vi "Plotter_Competition_Main_backup.vi"() -> ()   [LabVIEW 2014]
doc: "Buggy_Competition Main.vi\nv4.0\nCode fior Jan 2012\n\nModified by D.Readman 1/12/2011 to 5/1/2012 \n- Replaced shift registers with FGV's.\n- Latched Switch function added.\n- Digital filtering on encoder inputs added."
uses:
  Controls/Plotter States.ctl
  <vilib>/Platform/TimedLoop/XDataNode/timing_clust.ctl
  <vilib>/Platform/TimedLoop/XDataNode/nitl_modes.ctl
  <vilib>/Platform/TimedLoop/XDataNode/wakeup.ctl
  <vilib>/FPGAPlugInAG/myRIO-1900/niLvFpga_Open_myRIO-1900.vi
  <vilib>/rvi/interface/nirviOpenFPGA/nirviOpenFPGA.xnode
  FPGA Bitfiles/Buggycompetition_FPGATarget2_AeroBuggyFPGA_9DbUQD1BP7s.lvbitx
  FPGA/FPGA.vi
  <vilib>/Platform/TimedLoop/XDataNode/XDataNode.xnode
  <vilib>/Platform/TimedLoop/XDataNode/XDNodeRunTimeDep.lvlib
panel:
  out "Finished Late? [i-1]":bool
  in  "Sample interval":u32=100000
  in  "MWidth":i64=4
  out "Current State":T1
  out "Switch B":bool
  out "Switch A":bool
  in  "Enc. Filter":i16=2 min=0 step=1
  out "Switches Latched":cluster{"Switch A GN":bool, "Switch B BL":bool}
  in  "Terminate":bool
  out "Error Display":errorcluster
  in  "Reset Button":bool
  # "Impeccable Plotter Controller"
  # "Switches"
  # "Admin controls - Do not alter"
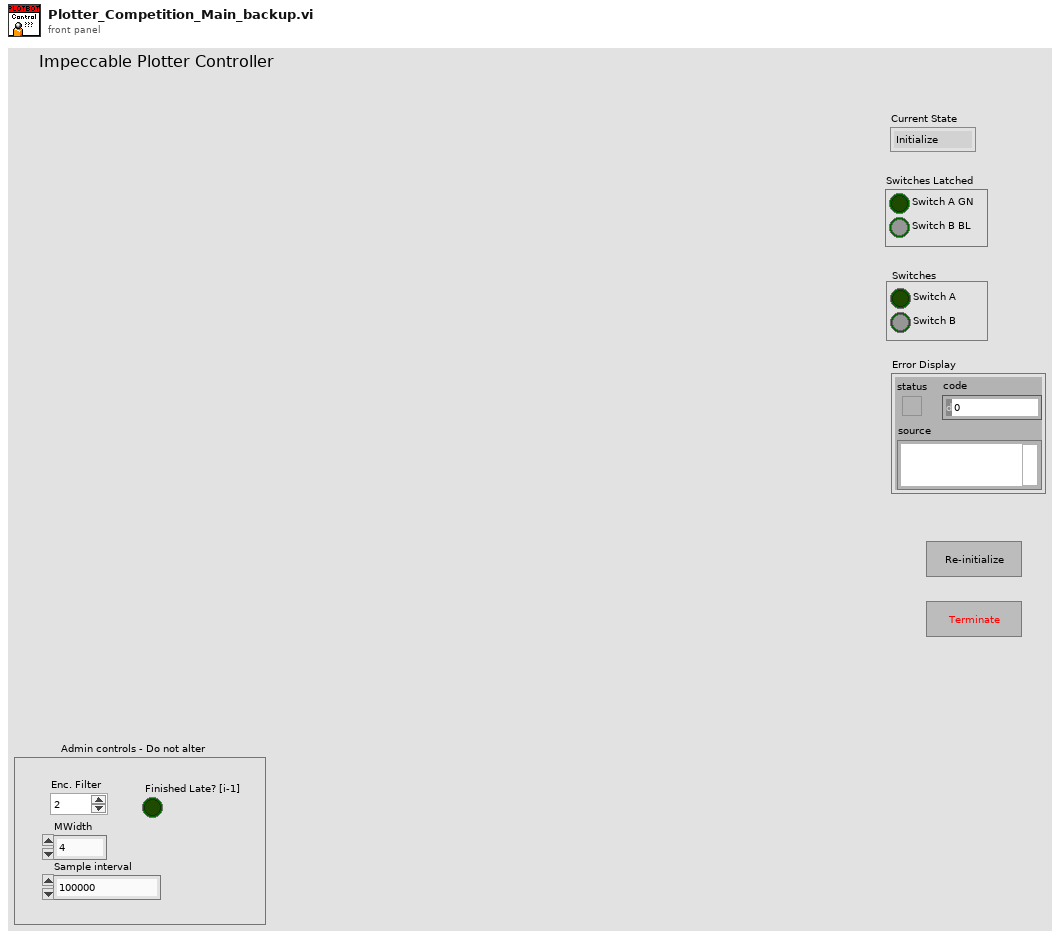
[diagram p1: front panel]
types:
  T1 = typedef "Plotter States.ctl" = enum16{"Initialize", "Run", "Stop"}
  T2 = cluster{"Data":dbl[], "Operation":enum16{"New folder/file", "Create file", "Record", "Close"}, "File name":string}
  T3 = typedef "XDNodeRunTimeDep.lvlib/timing_clust.ctl" = cluster{"Expected End [f-1]":u64, "Actual End [f-1]":u64, "Finished Late? [f-1]":bool, "Expected End [i-1]":u64, "Actual End [i-1]":u64, "Finished Late? [i-1]":bool, "Expected Start [i]":u64, "Actual Start [i]":u64, "Expected Start [f]":u64, "Actual Start [f]":u64, "Source Name":string, "Structure Name":string, "Period":i64, "Deadline":i64, "Offset":i64, "Start":i64, "Priority":i32, "Timeout":i32, "Mode":T4, "Wakeup Reason":T5, "Error":errorcluster, "Source Type":string, "Secondary Source Type":string, "Global End Time":u64, "Global Start Time":u64, "Frame Duration":u64, "Iteration Duration":u64, "Assigned CPU":i32, "I/O Scan Engine Mode":u32}
  T4 = typedef "XDNodeRunTimeDep.lvlib/nitl_modes.ctl" = enum32{"No Change", "Process missed periods, maintain original phase", "Discard missed periods, maintain original phase", "Process missed periods, ignore original phase", "Discard missed periods, ignore original phase"}
  T5 = typedef "XDNodeRunTimeDep.lvlib/wakeup.ctl" = enum32{"Normal", "Aborted", "Asynchronous wakeup", "Timing source error", "Timed loop error", "Timeout"}
  T6 = enum16{"New folder/file", "Create file", "Record", "Close"}
  T7 = cluster{"appended array":dbl[], "Operation":enum16{"New folder/file", "Create file", "Record", "Close"}, string}
  T8 = cluster{dbl[], "Operation":enum16{"New folder/file", "Create file", "Record", "Close"}, string}
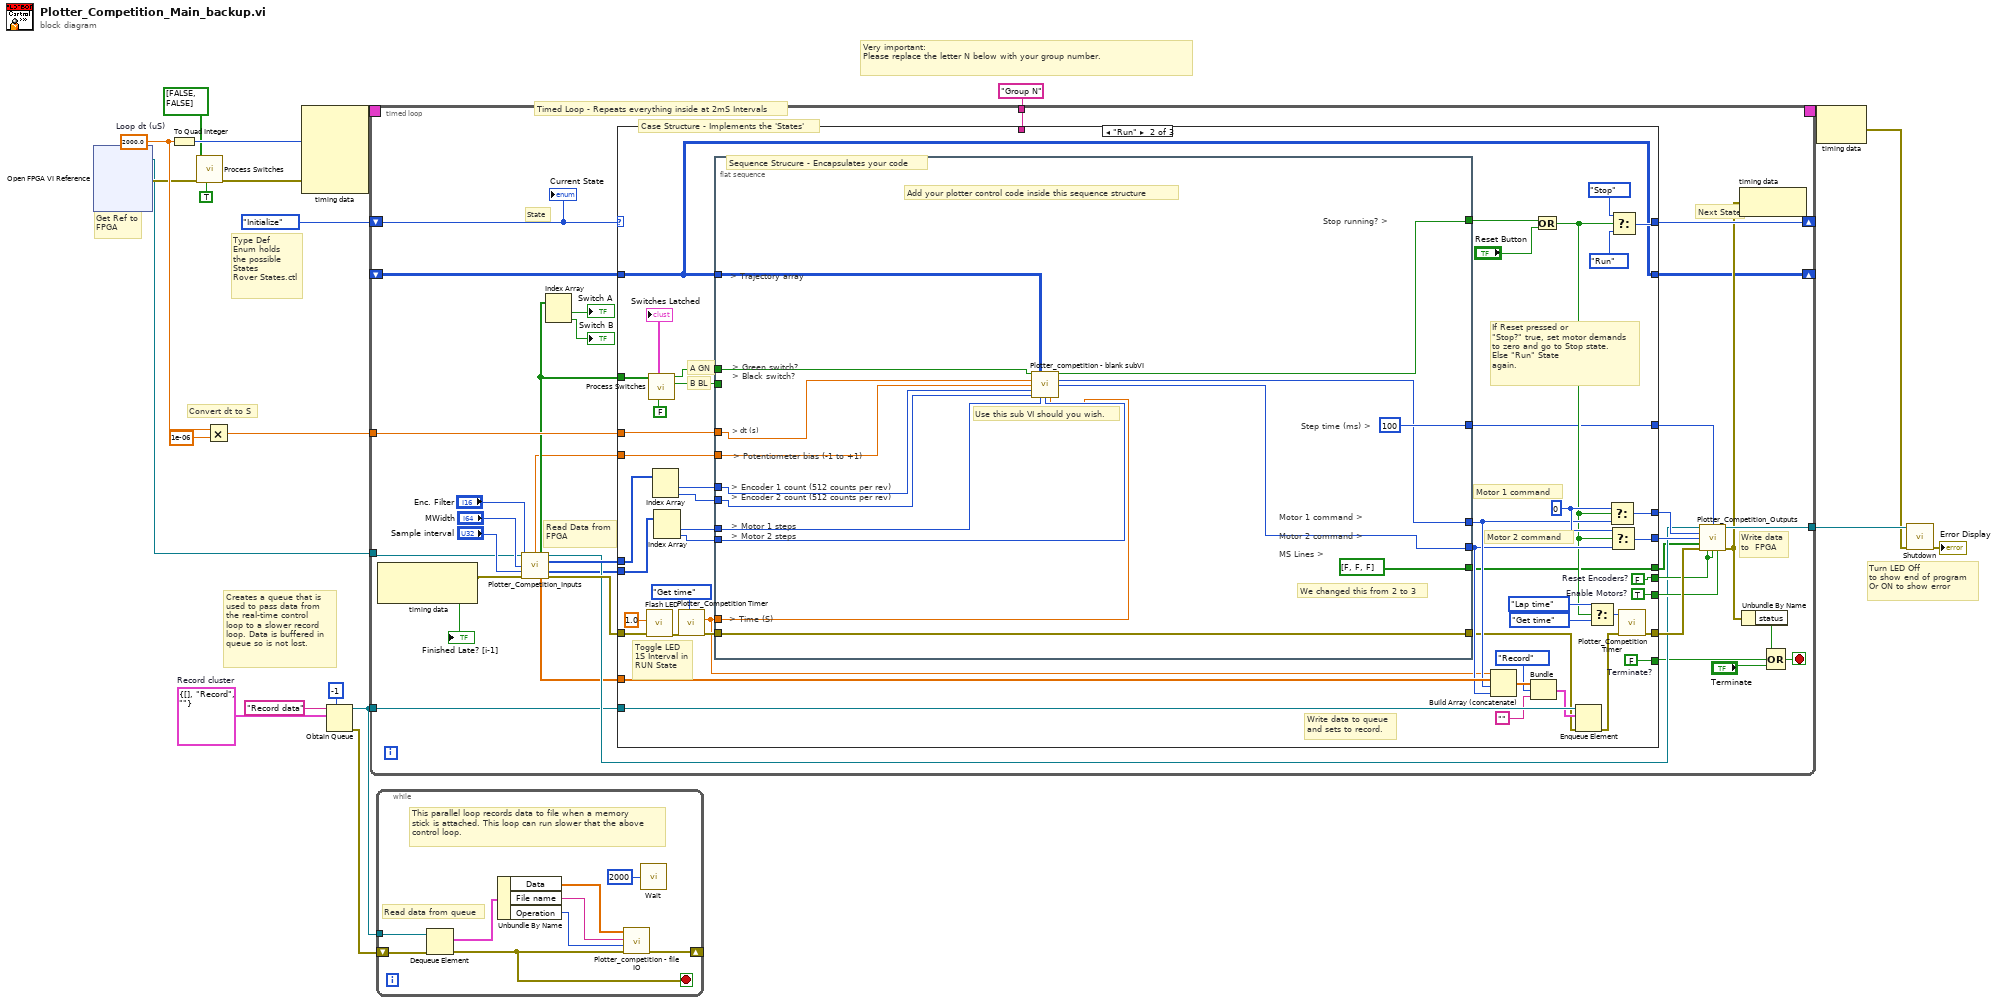
[diagram p0: block diagram]
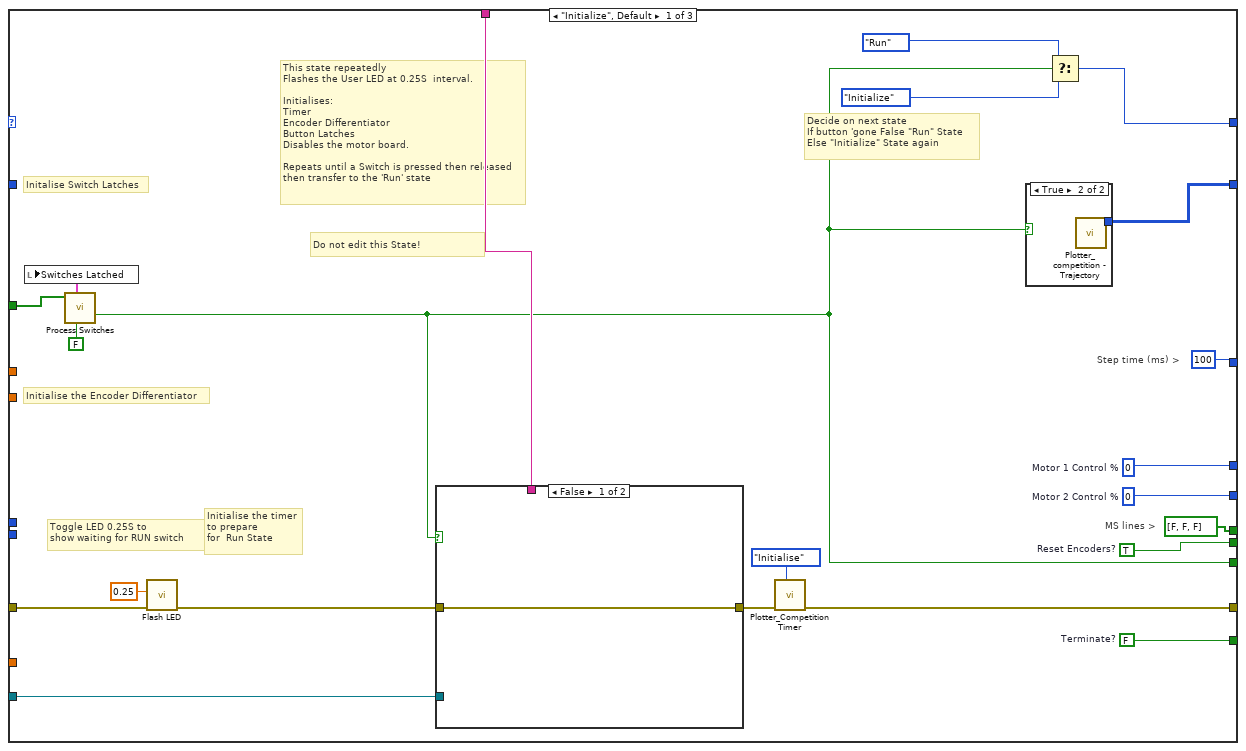
[diagram p2: hidden frame]
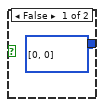
[diagram p3: hidden frame]
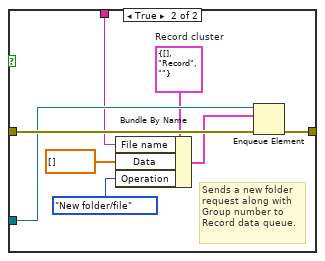
[diagram p4: hidden frame]
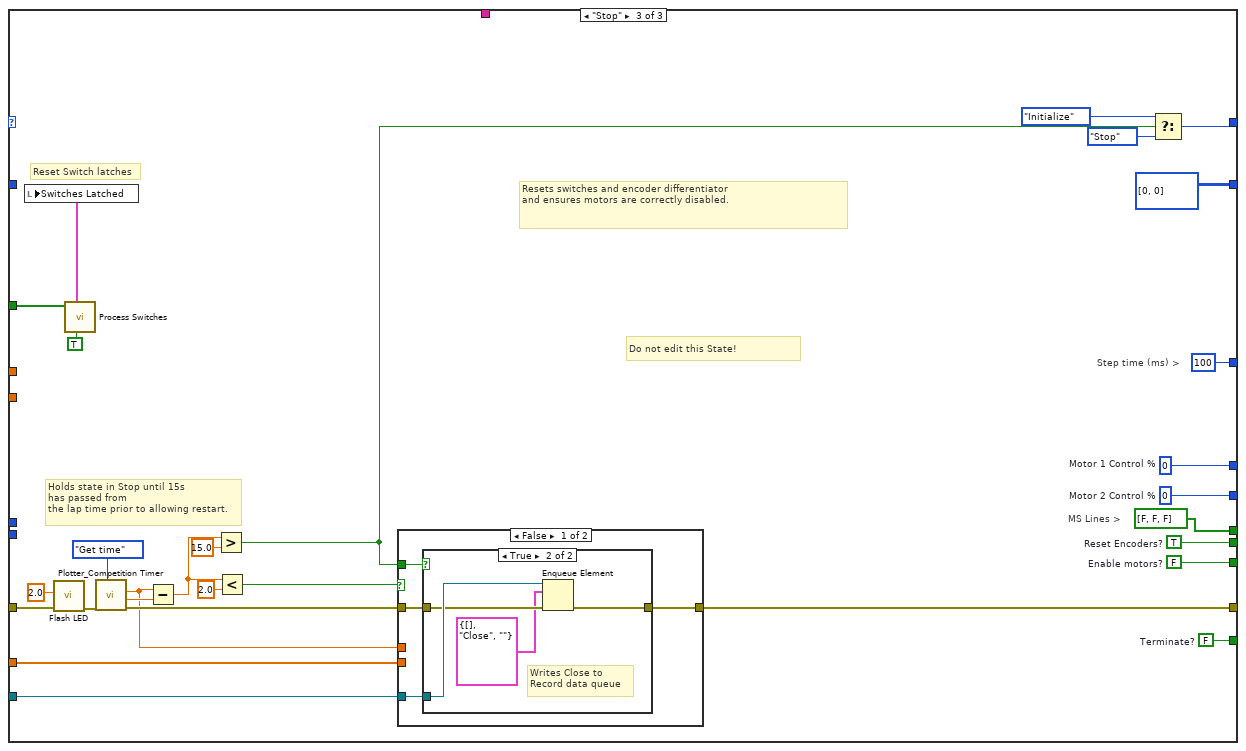
[diagram p5: hidden frame]
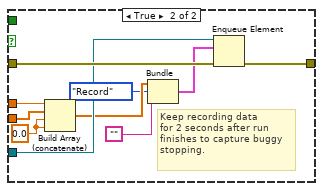
[diagram p7: hidden frame]
diagram:
  w6 = T2 {"Data"=[], "Operation"=enum."Record", "File name"=""}  # Record cluster
  w14 = 2000.0  # Loop dt (uS)
  # "Creates a queue that is\nused to pass data from\nthe real-time control \nloop to a slower record\nloop. Data is buffered in \nqueue so is not lost."
  # "Very important:\nPlease replace the letter N below with your group number."
  # "Type Def\nEnum holds\nthe possible\nStates\nRover States.ctl"
  # "Get Ref to\nFPGA"
  # "Timed Loop - Repeats everything inside at 2mS Intervals"
  # "Convert dt to S"
  # "Turn LED Off\nto show end of program\nOr ON to show error"
  n1 = xnode "Open FPGA VI Reference"() -> ("FPGA VI Reference Out"=w1:refnum<k20>, "error out"=w11:errorcluster)  [unwired: 2 in]
  n2 = To Quad Integer(1:w14) -> (0:w17:i64)
  n3 = call "Process Switches .vi"("Initialise?"=TRUE, "Error In"=w11, "Switches in"=bool[] [FALSE, FALSE]) -> ("Error Out"=w7:errorcluster)  [unwired: 4 in, 4 out]
  n4 = Multiply(x=w14, y=1e-06) -> (x*y=w12:dbl)
  n5 = node-c288(w17, w7) -> (w20:T3)  [unwired: 3 in]
  n6 = Obtain Queue(max queue size (-1, unlimited)=-1, name (unnamed)="Record data", element data type=w6) -> (queue out=w4:refnum<queue>, error out=w3:errorcluster)  [unwired: 2 in, 1 out]
  n7 = timed-loop {
    shift-right: [w55] -> _
    shift-left: Plotter_States."Initialize" ("Initial State") -> [w56]
    timing: w20 -> [_]
    timing-out: [_] -> w19
    tunnel: [w51] -> w18
    tunnel: w12 -> [w46]
    tunnel: w1 -> [w26]
    tunnel: "Group N" -> [w34]
    tunnel: w4 -> [w28]
    shift-right: [w23] -> _
    shift-left: _ -> [w22]
    stop <- w41 stop-if-true
    # "Case Structure - Implements the 'States'"
    # "Next State"
    # "Write data\nto  FPGA"
    # "Read Data from\nFPGA"
    # "State"
    n8 = node-c288() -> (w44:errorcluster, →"Finished Late? [i-1]":bool)  [unwired: 1 in]
    n9 = call "Plotter_Competition_Inputs.vi"("FPGA VI Reference"=w26, "Filter Iterations"="Enc. Filter", "Measurement Width (Counts)"="MWidth", "Max sample interval (uS)"="Sample interval", "Error In"=w44) -> ("Bias (-1 to +1)"=w27:dbl, "Switches Green or Black"=w31:bool[], "FPGA VI Reference Out"=w45:refnum<k20>, "Encoder count"=w54:i64[], "Motor Steps"=w35:i16[], "Data array"=w30:dbl[], "Error Out"=w53:errorcluster)  [unwired: 3 in, 1 out]
    n10 = Index Array(array=w31) -> (element #1=→"Switch A":bool, element #2=→"Switch B":bool)  [unwired: 2 in]
    n11 = case shown="\"Run\"" w56 {
      tunnel: [w84 w143 w179] -> w55
      tunnel: [w83 w139 w183] -> w42
      tunnel: w54 -> [_ w100 _]
      tunnel: w53 -> [w69 w104 w164]
      tunnel: [w72 w127 w175] -> w52
      tunnel: [w64 w140 w184] -> w50
      tunnel: [w82 w141 w185] -> w49
      tunnel: [w81 w135 w186] -> w48
      tunnel: [w80 w134 w187] -> w47
      tunnel: w46 -> [_ w128 _]
      tunnel: w35 -> [_ w123 _]
      tunnel: w34 -> [w75 _ _]
      tunnel: w31 -> [w74 w126 w173]
      tunnel: w30 -> [_ w120 w169]
      tunnel: w28 -> [w71 w116 w172]
      tunnel: w27 -> [_ w99 _]
      tunnel: [bool[] [FALSE, FALSE, FALSE] ("MS lines") w98 bool[] [FALSE, FALSE, FALSE] ("MS lines")] -> w25
      tunnel: [u32 100 ("Step time") w97 u32 100 ("Step time")] -> w24
      tunnel: [w63 w96 i32[][] [[0, 0]] ("Array")] -> w23
      tunnel: w22 -> [_ w96 _]
      frame "Initialize", Default {
        w80 = i8 0  # Motor 2 Control %
        w81 = i8 0  # Motor 1 Control %
        w82 = TRUE  # Reset Encoders?
        w83 = FALSE  # Terminate?
        # "MS lines >"
        # "Step time (ms) >"
        # "Initalise Switch Latches"
        # "Initialise the Encoder Differentiator"
        # "This state repeatedly\nFlashes the User LED at 0.25S  interval.\n\nInitialises:\nTimer\nEncoder Differentiator\nButton Latches\nDisables the motor board.\n\nRepeats until a Switch is pressed then released\nthen transfer to the 'Run' state"
        # "Initialise the timer\nto prepare\nfor  Run State"
        # "Toggle LED 0.25S to\nshow waiting for RUN switch"
        # "Do not edit this State!"
        # "Decide on next state\nIf button 'gone False \"Run\" State\nElse \"Initialize\" State again"
        n12 = call "Process Switches .vi"("Initialise?"=FALSE, "Switches in"=w74) -> ("Switch Released?"=w64:bool, "Switches Latched Cluster"=w78:cluster{"Switch A GN":bool, "Switch B BL":bool})  [unwired: 5 in, 3 out]
        n13 = local write "Switches Latched"(w78) -> ()
        n14 = call "Flash LED.vi"("Error In"=w69, "Interval (S) (1 S)"=0.25) -> ("Error Out"=w68:errorcluster)  [unwired: 8 in, 1 out]
        n15 = case shown="False" w64 {
          tunnel: w68 -> [w87 w95]
          tunnel: [w87 w94] -> w73
          tunnel: w75 -> [_ w90]
          tunnel: w71 -> [_ w93]
          frame False {
          }
          frame True {
            w91 = T2 {"Data"=[], "Operation"=enum."Record", "File name"=""}  # Record cluster
            # "Sends a new folder\nrequest along with\nGroup number to \nRecord data queue."
            n16 = Bundle By Name(cluster=w91, "File name"=w90, "Data"=dbl[] [] ("appended array"), "Operation"=T6."New folder/file") -> (w92:T2)
            n17 = Enqueue Element(queue=w93, element=w92, error in (no error)=w95) -> (error out=w94:errorcluster)  [unwired: 1 in, 2 out]
          }
        }
        n18 = call "Plotter_Competition Timer.vi"("Timer state"=enum16{"Initialise", "Get time", "Lap time"}."Initialise", "Error In"=w73) -> ("Error Out"=w72:errorcluster)  [unwired: 7 in, 2 out]
        n19 = case shown="True" w64 {
          tunnel: [i32[][] [[0, 0]] ("Array") w86] -> w63
          frame False {
          }
          frame True {
            n20 = call "Plotter_competition - Trajectory.vi"() -> ("Array"=w86:i32[][])  [unwired: 11 in]
          }
        }
        n21 = Select(t=Plotter_States."Run" ("Buggy State"), s=w64, f=Plotter_States."Initialize" ("Buggy State")) -> (s? t:f=w84:T1)
      }
      frame "Run" {
        w133 = i8 0 ("t")
        w139 = FALSE  # Terminate?
        w140 = TRUE  # Enable Motors?
        w141 = FALSE  # Reset Encoders?
        # "Write data to queue\nand sets to record."
        # "If Reset pressed or\n\"Stop?\" true, set motor demands\nto zero and go to Stop state.\nElse \"Run\" State\nagain."
        # "B BL"
        # "A GN"
        # "Sequence Strucure - Encapsulates your code"
        # "Motor 2 command"
        # "Motor 1 command"
        # "Toggle LED\n1S Interval in\nRUN State"
        n22 = call "Flash LED.vi"("Error In"=w104, "Interval (S) (1 S)"=1.0) -> ("Error Out"=w103:errorcluster)  [unwired: 8 in, 1 out]
        n23 = call "Process Switches .vi"("Initialise?"=FALSE, "Switches in"=w126) -> ("Switch B Latched"=w137:bool, "Switch A Latched"=w138:bool, "Switches Latched Cluster"=→"Switches Latched":cluster{"Switch A GN":bool, "Switch B BL":bool})  [unwired: 5 in, 2 out]
        n24 = Index Array(array=w100) -> (element #1=w125:i64, element #2=w124:i64)  [unwired: 2 in]
        n25 = Index Array(array=w123) -> (element #1=w122:i16, element #2=w121:i16)  [unwired: 2 in]
        n26 = call "Plotter_Competition Timer.vi"("Timer state"=enum16{"Initialise", "Get time", "Lap time"}."Get time", "Error In"=w103) -> ("Error Out"=w142:errorcluster, "Elapsed Time Out (S)"=w117:dbl)  [unwired: 7 in, 1 out]
        n27 = flat-sequence {
          tunnel: [w151] -> w119
          tunnel: [w150] -> w118
          tunnel: w142 -> [w158]
          tunnel: [w158] -> w112
          tunnel: w117 -> [w144]
          tunnel: w138 -> [w149]
          tunnel: w137 -> [_]
          tunnel: w128 -> [w152]
          tunnel: w125 -> [w154]
          tunnel: w124 -> [w153]
          tunnel: w122 -> [w147]
          tunnel: w121 -> [w146]
          tunnel: [w145] -> w101
          tunnel: w99 -> [w148]
          tunnel: [bool[] [FALSE, FALSE, FALSE] ("MS lines")] -> w98
          tunnel: [u32 100 ("Step time")] -> w97
          tunnel: w96 -> [w155]
          frame #0 {
            # "We changed this from 2 to 3"
            # "> Trajectory array"
            # "Step time (ms) >"
            # "Use this sub VI should you wish."
            # "Motor 1 command >\n\nMotor 2 command >\n\nMS Lines >"
            # "Stop running? >"
            # "> Green switch?\n> Black switch?"
            # "> dt (s)"
            # "> Potentiometer bias (-1 to +1)"
            # "> Encoder 1 count (512 counts per rev)\n> Encoder 2 count (512 counts per rev)"
            # "> Motor 1 steps\n> Motor 2 steps"
            # "Add your plotter control code inside this sequence structure"
            # "> Time (S)"
            n28 = call "Plotter_competition - blank subVI.vi"("Switch A Latched"=w149, "Array"=w155, "dt in sec"=w152, "Potentiometer bias (-1 to +1)"=w148, "Encoder 1 count"=w154, "Encoder 2 count"=w153, "Motor steps 1"=w147, "Motor steps 2"=w146, "Elapsed Time Out (S)"=w144) -> ("Stop"=w145:bool, "Motor 1 command"=w151:i8, "Motor 2 command"=w150:i8)  [unwired: 3 in, 1 out]
          }
        }
        n29 = Build Array (concatenate)(w117, w120, w119, w118) -> (w114:dbl[])
        n30 = Bundle(w114, "Operation"=T6."Record", "") -> (w115:T8)  [unwired: 1 in]
        n31 = Or(x=w101, y="Reset Button") -> (x .or. y?=w106:bool)
        n32 = Enqueue Element(queue=w116, element=w115, error in (no error)=w112) -> (error out=w111:errorcluster)  [unwired: 1 in, 2 out]
        n33 = Select(t=enum16{"Initialise", "Get time", "Lap time"}."Lap time" ("Timer state"), s=w106, f=enum16{"Initialise", "Get time", "Lap time"}."Get time" ("Timer state")) -> (s? t:f=w108:enum16{"Initialise", "Get time", "Lap time"})
        n34 = Select(t=w133, s=w106, f=w119) -> (s? t:f=w135:i8)
        n35 = Select(t=w133, s=w106, f=w118) -> (s? t:f=w134:i8)
        n36 = Select(t=Plotter_States."Stop" ("Buggy State"), s=w106, f=Plotter_States."Run" ("Buggy State")) -> (s? t:f=w143:T1)
        n37 = call "Plotter_Competition Timer.vi"("Timer state"=w108, "Error In"=w111) -> ("Error Out"=w127:errorcluster)  [unwired: 7 in, 2 out]
      }
      frame "Stop" {
        w183 = FALSE  # Terminate?
        w184 = FALSE  # Enable motors?
        w185 = TRUE  # Reset Encoders?
        w186 = i8 0  # Motor 1 Control %
        w187 = i8 0  # Motor 2 Control %
        # "MS Lines >"
        # "Step time (ms) >"
        # "Holds state in Stop until 15s\nhas passed from\nthe lap time prior to allowing restart."
        # "Resets switches and encoder differentiator\nand ensures motors are correctly disabled."
        # "Do not edit this State!"
        # "Reset Switch latches"
        n38 = call "Flash LED.vi"("Error In"=w164, "Interval (S) (1 S)"=2.0) -> ("Error Out"=w163:errorcluster)  [unwired: 8 in, 1 out]
        n39 = call "Process Switches .vi"("Initialise?"=TRUE, "Switches in"=w173) -> ("Switches Latched Cluster"=w181:cluster{"Switch A GN":bool, "Switch B BL":bool})  [unwired: 5 in, 4 out]
        n40 = local write "Switches Latched"(w181) -> ()
        n41 = call "Plotter_Competition Timer.vi"("Timer state"=enum16{"Initialise", "Get time", "Lap time"}."Get time", "Error In"=w163) -> ("Error Out"=w176:errorcluster, "Lap time out (s)"=w167:dbl, "Elapsed Time Out (S)"=w165:dbl)  [unwired: 7 in]
        n42 = Subtract(x=w165, y=w167) -> (x-y=w166:dbl)
        n43 = Greater?(x=w166, y=15.0) -> (0:w174:bool)
        n44 = Less?(x=w166, y=2.0) -> (x < y?=w170:bool)
        n45 = case shown="False" w170 {
          tunnel: w176 -> [w191 w206]
          tunnel: [w190 w205] -> w175
          tunnel: w174 -> [w189 _]
          tunnel: w172 -> [w188 w204]
          tunnel: w169 -> [_ w198]
          tunnel: w165 -> [_ w203]
          frame False {
            n46 = case shown="True" w189 {
              tunnel: w191 -> [w192 w195]
              tunnel: [w192 w194] -> w190
              tunnel: w188 -> [_ w196]
              frame False {
              }
              frame True {
                # "Writes Close to \nRecord data queue"
                n47 = Enqueue Element(queue=w196, element=T7 {"appended array"=[], "Operation"=enum."Close", ""}, error in (no error)=w195) -> (error out=w194:errorcluster)  [unwired: 1 in, 2 out]
              }
            }
          }
          frame True {
            w197 = 0.0 ("y")
            # "Keep recording data\nfor 2 seconds after run\nfinishes to capture buggy\nstopping."
            n48 = Build Array (concatenate)(w203, w198, w197, w197) -> (w202:dbl[])
            n49 = Bundle(w202, "Operation"=T6."Record", "") -> (w199:T8)  [unwired: 1 in]
            n50 = Enqueue Element(queue=w204, element=w199, error in (no error)=w206) -> (error out=w205:errorcluster)  [unwired: 1 in, 2 out]
          }
        }
        n51 = Select(t=Plotter_States."Initialize" ("Buggy State"), s=w174, f=Plotter_States."Stop") -> (s? t:f=w179:T1)
      }
    }
    n52 = call "Plotter_Competition_Outputs.vi"("FPGA VI Reference"=w45, "Step time"=w24, "Motor 1 command"=w48, "Motor 2 command"=w47, "MS lines"=w25, "Error In"=w52, "Reset encoder 1?"=w49, "Reset encoder 2?"=w49, "Enable motors?"=w50) -> ("FPGA VI Reference out"=w51:refnum<k20>, "Error Out"=w39:errorcluster)  [unwired: 5 in]
    n53 = node-c288(w39) -> ()  [unwired: 1 out]
    n54 = Unbundle By Name(w39) -> ("status"=w43:bool)
    n55 = Compound Arithmetic op=OR(w43, w42, "Terminate") -> (w41:bool)
    "Current State" <- w56
  }
  n56 = while {
    tunnel: w4 -> [w215]
    shift-right: [w210] -> _
    shift-left: w3 -> [w214]
    stop <- w211 stop-if-true
    # "Read data from queue"
    # "This parallel loop records data to file when a memory\nstick is attached. This loop can run slower that the above\ncontrol loop."
    n57 = Dequeue Element(queue=w215, error in (no error)=w214) -> (element=w213:T2, error out=w211:errorcluster)  [unwired: 1 in, 2 out]
    n58 = Unbundle By Name(w213) -> ("Data"=w212:dbl[], "File name"=w208:string, "Operation"=w207:T6)
    n59 = call "Plotter_competition - file IO.vi"("error in"=w211, "Operation"=w207, "File name"=w208, "Data"=w212) -> ("error out"=w210:errorcluster)  [unwired: 7 in]
    n60 = call "Wait"("Count(uSec)"=u32 2000) -> ()  [unwired: 1 out]
  }
  n61 = node-c288(w19) -> (w16:errorcluster)
  n62 = call "Shutdown.vi"("Error"=w16, "FPGA VI Reference"=w18) -> ("Error Display"=→"Error Display":errorcluster)  [unwired: 8 in]
